vi "Recall Setup.vi"(8 "error in (no error)":errorcluster, 9 "File Name (seup_9)":string="setup_9", 10 "Working Directory (\\Agilent Flash\\setups\\)":string="\\Agilent Flash\\setups\\", 11 "VISA resource name":refnum<visa-resource-name>="MSO") -> (0 "error out":errorcluster, 3 "VISA resource name out":refnum<visa-resource-name>="MSO")   [LabVIEW 2015, in "Agilent 2000 3000 X-Series.lvlib"]
doc: "Recalls previously saved oscilloscope setups, waveforms, and masks."
uses:
  Agilent 2000 3000 X-Series.lvlib
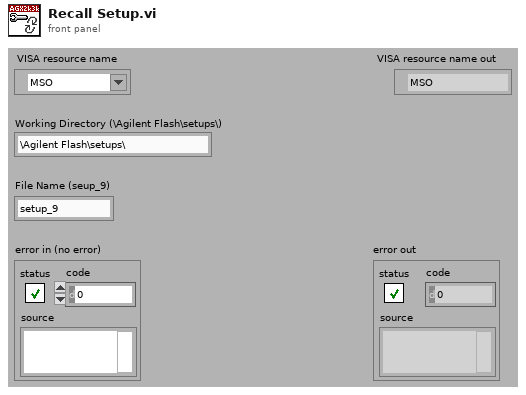
[diagram p1: front panel]
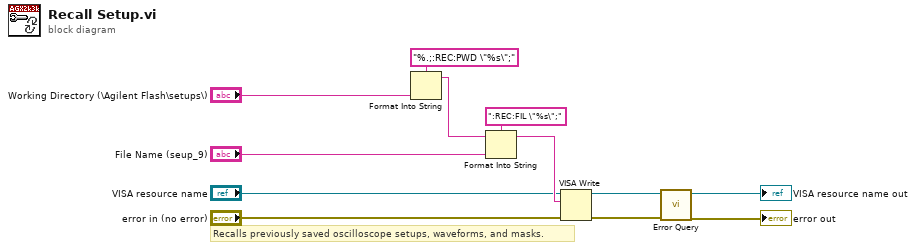
[diagram p0: block diagram]
diagram:
  # "Recalls previously saved oscilloscope setups, waveforms, and masks."
  n1 = Format Into String(format string="%.;:REC:PWD \"%s\";", "Working Directory (\\Agilent Flash\\setups\\)") -> (resulting string=w10:string)  [unwired: 2 in, 1 out]
  n2 = Format Into String(format string=":REC:FIL \"%s\";", initial string=w10, "File Name (seup_9)") -> (resulting string=w7:string)  [unwired: 1 in, 1 out]
  n3 = VISA Write(VISA resource name="VISA resource name", write buffer=w7, error in (no error)="error in (no error)") -> (VISA resource name out=w4:refnum<visa-resource-name>, error out=w3:errorcluster)  [unwired: 1 out]
  n4 = call "Error Query.vi"("error in (no error)"=w3, "VISA resource name"=w4) -> ("error out"=→"error out":errorcluster, "VISA resource name out"=→"VISA resource name out":refnum<visa-resource-name>)  [unwired: 8 out]
